vi "Servo Math.vi"(9 "upper limit":dbl=254.0 format="%#_13g", 10 "Multipy Factor":dbl=3.0 format="%#_13g", 11 "X axis rotation":dbl) -> (3 "Numeric":dbl)   [LabVIEW 2018]
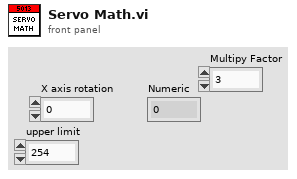
[diagram p1: front panel]
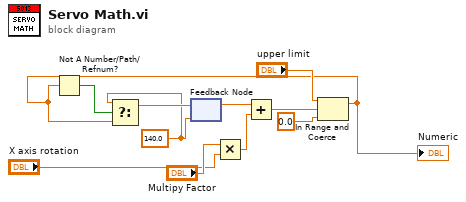
[diagram p0: block diagram]
diagram:
  w1 = 140.0
  n1 = feedback #1(w1) -> (w5:dbl)
  n2 = Multiply(x="Multipy Factor", y="X axis rotation") -> (x*y=w10:dbl)
  n3 = Add(x=w5, y=w10) -> (x+y=w11:dbl)
  n4 = In Range and Coerce(upper limit="upper limit", x=w11, lower limit=0.0) -> (coerced(x)=w2:dbl)  [unwired: 1 out]
  "Numeric" <- w2
  n5 = Not A Number/Path/Refnum?(number/path/refnum=w2) -> (NaN/Path/Refnum?=w3:bool)
  n6 = Select(t=w1, s=w3, f=w2) -> (s? t:f=w4:dbl)
  n7 = feedback-in #1(w4) -> ()
